vi "Cartesian Matrix 2 2D Array.vi"(10 "Matrix In":T2) -> (2 "Matrix Out":T1)   [LabVIEW 2013]
uses:
  Metadata/Cartesian Matrix.ctl
  Metadata/Cartesian Point.ctl
  Control Loop/Limit Matrix.ctl
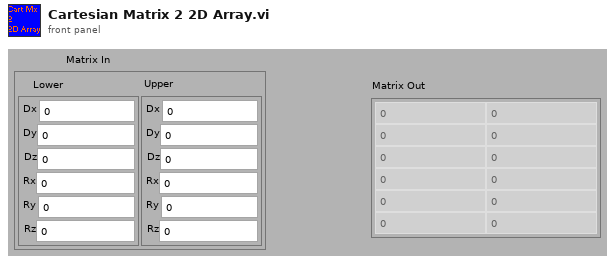
[diagram p1: front panel]
types:
  T1 = typedef "Limit Matrix.ctl" = dbl[][]
  T2 = typedef "Cartesian Matrix.ctl" = cluster{"Lower":T3, "Upper":T3}
  T3 = typedef "Cartesian Point.ctl" = cluster{"Dx":dbl, "Dy":dbl, "Dz":dbl, "Rx":dbl, "Ry":dbl, "Rz":dbl}
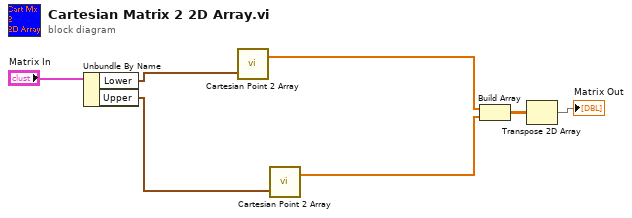
[diagram p0: block diagram]
diagram:
  n1 = Unbundle By Name("Matrix In") -> ("Lower"=w6:T3, "Upper"=w3:T3)
  n2 = call "Cartesian Point 2 Array.vi"("Cart Disp"=w6) -> ("Array"=w2:dbl[])  [unwired: 2 out]
  n3 = call "Cartesian Point 2 Array.vi"("Cart Disp"=w3) -> ("Array"=w1:dbl[])  [unwired: 2 out]
  n4 = Build Array(w2, w1) -> (w5:dbl[][])
  n5 = Transpose 2D Array(2D array=w5) -> (transposed array=→"Matrix Out":dbl[][])
